vi "Write Contour Display Rate (SubVI).vi"(11 "Rate (Hz)":u32) -> ()   [LabVIEW 2020]
uses:
  <vilib>/Utility/config.llb/Write Key (U32).vi
  <vilib>/Utility/config.llb/NI_LVConfig.lvlib
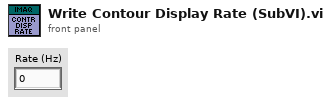
[diagram p1: front panel]
types:
  T1 = typedef "NI_LVConfig.lvlib/Config Data RefNum.ctl" = refnum<k1>
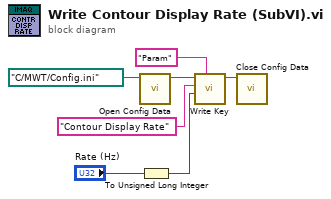
[diagram p0: block diagram]
diagram:
  n1 = call <vilib>:"Open Config Data.vi"("configuration file path"=path "C:/MWT/Config.ini") -> ("refnum"=w7:T1)  [unwired: 8 in, 2 out]
  n2 = To Unsigned Long Integer(number="Rate (Hz)") -> (unsigned 32bit integer=w2:u32)
  n3 = call-poly <vilib>:"Write Key.vi"("section"="Param", "value"=w2, "key"="Contour Display Rate" ("section"), "refnum"=w7) -> ("refnum out"=w5:T1)  [unwired: 5 in, 2 out]
  n4 = call <vilib>:"Close Config Data.vi"("refnum"=w5) -> ()  [unwired: 9 in, 2 out]
